vi "statesSeperator.vi"(10 "q":dbl[](array[numeric])) -> (0 "q2 dq2":T1, 1 "q1 dq1":T1, 2 "vel dq":T1, 3 "pos q":T1)   [LabVIEW 2019]
uses:
  <vilib>/Analysis/Matrix/Datatypes/RealMatrix.ctl
  <vilib>/Analysis/Matrix/NI_Matrix.lvlib
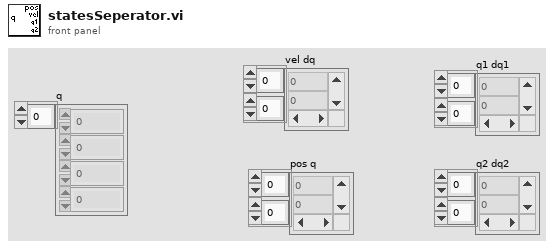
[diagram p1: front panel]
types:
  T1 = typedef "NI_Matrix.lvlib/RealMatrix.ctl" = dbl[][]
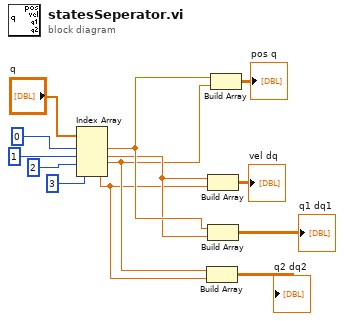
[diagram p0: block diagram]
diagram:
  n1 = Index Array(array="q", index #1=0 ("index (row)"), index #2=1 ("index (col)"), index #3=2 ("index"), index #4=3 ("index")) -> (element #1=w6:dbl, element #2=w5:dbl, element #3=w3:dbl, element #4=w2:dbl)
  n2 = Build Array(w3, w2) -> (→"q2 dq2":T1)
  n3 = Build Array(w5, w2) -> (→"vel dq":T1)
  n4 = Build Array(w6, w5) -> (→"q1 dq1":T1)
  n5 = Build Array(w6, w3) -> (→"pos q":T1)
